vi "Remove Tasks.vi"(8 "error in (no error)":errorcluster, 10 "User Selections":i32[](array[numeric]), 11 "BuildServer in":refnum<class "BuildServer.lvclass">) -> (0 "error out":errorcluster, 3 "BuildServer out":refnum<class "BuildServer.lvclass">)   [LabVIEW 2017, in "BuildServer.lvlib" / "BuildServer.lvclass"]
uses:
  BuildServer.lvclass
  C:/Program Files (x86)/National Instruments/LabVIEW 2017/vi.lib/ActorFramework/Actor/Actor.lvclass
  <vilib>/ActorFramework/Actor/Actor.lvclass/Actor.ctl
  <vilib>/ActorFramework/Message Enqueuer/Message Enqueuer.lvclass/Message Enqueuer.ctl
  <vilib>/ActorFramework/Message Enqueuer/Init from Existing Queue.vi
  <vilib>/ActorFramework/Message Enqueuer/Enqueue.vi
  BuildServer Messages/Update TaskView Msg/Update TaskView Msg.lvclass
  C:/Program Files (x86)/National Instruments/LabVIEW 2017/vi.lib/ActorFramework/Message/Message.lvclass
  <vilib>/ActorFramework/Message Priority Queue/Priority Enqueue.vi
  <vilib>/ActorFramework/Message Enqueuer/Message Enqueuer.lvclass
  <vilib>/ActorFramework/Actor/Actor.lvclass
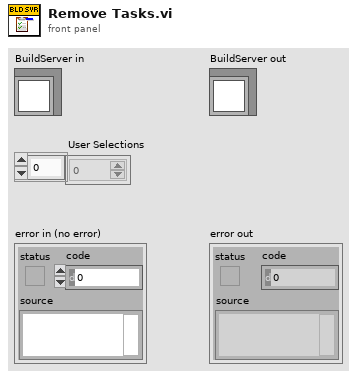
[diagram p1: front panel]
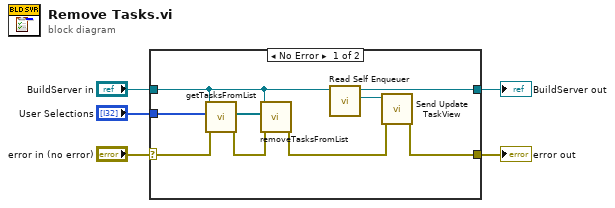
[diagram p0: block diagram]
diagram:
  n1 = case shown="No Error" "error in (no error)" {
    selector: "error in (no error)" -> [w9 w15]
    tunnel: [w11 w15] -> w4
    tunnel: [w10 w14] -> w2
    tunnel: "BuildServer in" -> [w10 w14]
    tunnel: "User Selections" -> [w6 _]
    frame No Error {
      n2 = call "getTasksFromList.vi"("error in (no error)"=w9, "User Selection"=w6, "BuildServer in"=w10) -> ("error out"=w8:errorcluster, "Selected Tasks"=w7:refnum<class "Task.lvclass">[])  [unwired: 7 in]
      n3 = call "removeTasksFromList.vi"("error in (no error)"=w8, "Selected Tasks"=w7, "BuildServer in"=w10) -> ("error out"=w12:errorcluster)  [unwired: 8 in]
      n4 = call <vilib>:"Read Self Enqueuer.vi"("Actor"=w10) -> ("Self Enqueuer"=w13:refnum<class "Message Enqueuer.lvclass">)  [unwired: 10 in]
      n5 = call "Send Update TaskView.vi"("error in (no error)"=w12, "Message Enqueuer in"=w13) -> ("error out"=w11:errorcluster)  [unwired: 8 in, 1 out]
    }
    frame Error {
    }
  }
  "error out" <- w4
  "BuildServer out" <- w2
